vi "Shutdown.vi"(8 "error in (no error)":errorcluster, 11 "Framework in":refnum<class "Framework.lvclass">) -> (0 "error out":errorcluster, 3 "Framework out":refnum<class "Framework.lvclass">)   [LabVIEW 2017, in "DSF Core.lvlib" / "Framework.lvclass"]
uses:
  Framework.lvclass
  Framework.lvclass/Framework.ctl
  Interfaces/Dispatcher/Command Data.ctl
  Interfaces/Dispatcher/Command.ctl
  Interfaces/Dispatcher/Parameters.ctl
  Interfaces/Interface/Interface.lvclass/Interface.ctl
  Debug/FIFO Flags/FIFO Flags.lvclass/FIFO Flags.ctl
  Interfaces/Dispatcher/Write Dispatcher Command.vi
  Interfaces/Interface/Write Command.vi
  Interfaces/Interface/Get Command FIFO.vi
  Interfaces/Interface/Write RT FIFO(16B).vi
  Interfaces/Interface/Get Debug Flags.vi
  Debug/FIFO Flags/Get Infinite Timeouts.vi
  Interfaces/Dispatcher/Dispatcher Interface.lvclass
  C:/Git/DSF/Data Sharing Framework/Source/Core/Engine/Classes/Interfaces/Interface/Interface.lvclass
  Interfaces/Interface/Errors.vi
  Interfaces/Interface/Command Timeout.vi
  Plugin/Plugin.lvclass
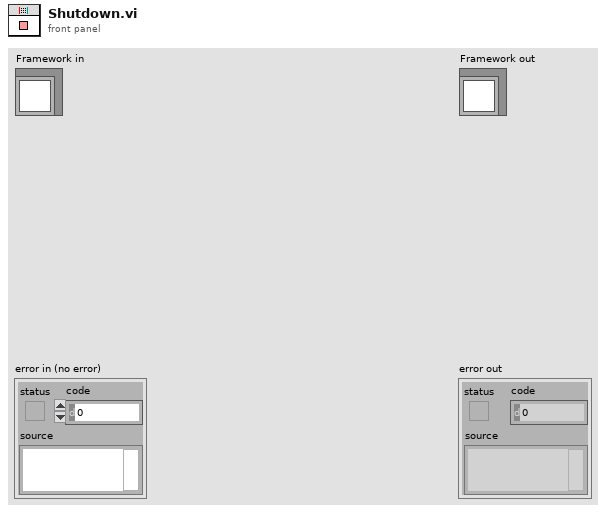
[diagram p1: front panel]
types:
  T1 = typedef "DSF Core.lvlib/Dispatcher Interface.lvclass/Command Data.ctl" = cluster{"Command":T2, "Parameters":T3}
  T2 = typedef "DSF Core.lvlib/Dispatcher Interface.lvclass/Command.ctl" = enum8{"Rx", "Tx", "Shutdown"}
  T3 = typedef "DSF Core.lvlib/Dispatcher Interface.lvclass/Parameters.ctl" = cluster{"arg1":u64, "arg2":u64}
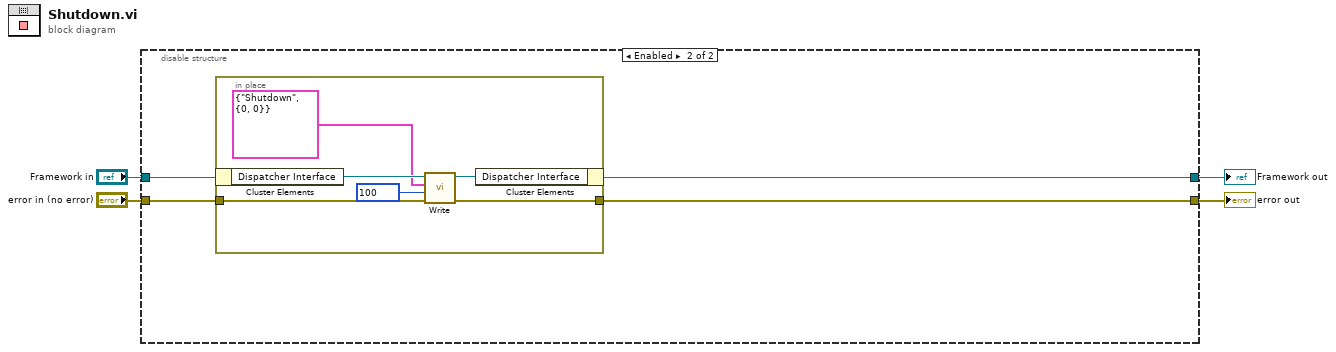
[diagram p0: block diagram]
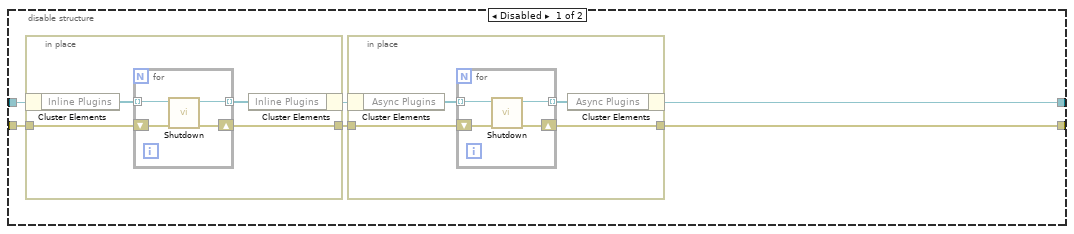
[diagram p2: hidden frame]
diagram:
  n1 = disable-structure shown="Enabled" {
    disable-tunnel: "error in (no error)" -> [w8 w29]
    disable-tunnel: "Framework in" -> [w7 w30]
    disable-tunnel: [w6 w28] -> w2
    disable-tunnel: [w5 w27] -> w1
    frame Disabled {
      n2 = in-place {
        in-place-border: w8 -> [w14]
        in-place-border: [w13] -> w10
        n3 = in-place-cluster #1(w7) -> ("Inline Plugins"=w12:refnum<class "Plugin.lvclass">[])
        n4 = for {
          tunnel: w12 -> [w15] mode=indexing
          tunnel: [w16] -> w11 mode=indexing
          shift-right: [w17] -> w13
          shift-left: w14 -> [w18]
          n5 = call "Shutdown.vi"("error in (no error)"=w18, "Plugin in"=w15) -> ("error out"=w17:errorcluster, "Plugin out"=w16:refnum<class "Plugin.lvclass">)  [unwired: 8 in]
        }
        n6 = in-place-cluster #1("Inline Plugins"=w11) -> (w9:refnum<class "Framework.lvclass">)
      }
      n7 = in-place {
        in-place-border: w10 -> [w22]
        in-place-border: [w21] -> w5
        n8 = in-place-cluster #2(w9) -> ("Async Plugins"=w20:refnum<class "Plugin.lvclass">[])
        n9 = for {
          tunnel: w20 -> [w23] mode=indexing
          tunnel: [w24] -> w19 mode=indexing
          shift-right: [w25] -> w21
          shift-left: w22 -> [w26]
          n10 = call "Shutdown.vi"("error in (no error)"=w26, "Plugin in"=w23) -> ("error out"=w25:errorcluster, "Plugin out"=w24:refnum<class "Plugin.lvclass">)  [unwired: 8 in]
        }
        n11 = in-place-cluster #2("Async Plugins"=w19) -> (w6:refnum<class "Framework.lvclass">)
      }
    }
    frame Enabled {
      n12 = in-place {
        in-place-border: w29 -> [w35]
        in-place-border: [w32] -> w27
        n13 = in-place-cluster #3(w30) -> ("Dispatcher Interface"=w36:refnum<class "Dispatcher Interface.lvclass">)
        n14 = call-poly "Write.vi"("error in (no error)"=w35, "timeout in ms (0)"=100, "command"=T1 {"Command"=enum."Shutdown", "Parameters"={"arg1"=0, "arg2"=0}}, "Dispatcher Interface in"=w36) -> ("error out"=w32:errorcluster, "Dispatcher Interface out"=w31:refnum<class "Dispatcher Interface.lvclass">)  [unwired: 5 in, 1 out]
        n15 = in-place-cluster #3("Dispatcher Interface"=w31) -> (w28:refnum<class "Framework.lvclass">)
      }
    }
  }
  "error out" <- w1
  "Framework out" <- w2
